vi "pid analog.vi"() -> ()   [LabVIEW 2015]
uses:
  <vilib>/addons/control/pid/pid.llb/PID Control Input Filter (DBL).vi
  <vilib>/addons/control/pid/pid.llb/PID (DBL).vi
  <vilib>/addons/control/pid/pid.llb/PID Output Rate Limiter (DBL).vi
  <vilib>/addons/control/pid/NI_PID_pid.lvlib
panel:
  in  "Array":dbl[](array[numeric])
  in  "Slide 2":dbl(slide) scale=0.0..10.0
  out "Waveform Chart":T1(graph)
  in  "stop":bool
  in  "output rate (EGU/min)":dbl=1.0 format="%.2f"
  in  "dt (s)":dbl=-1.0 format="%.3f"
  # "e"
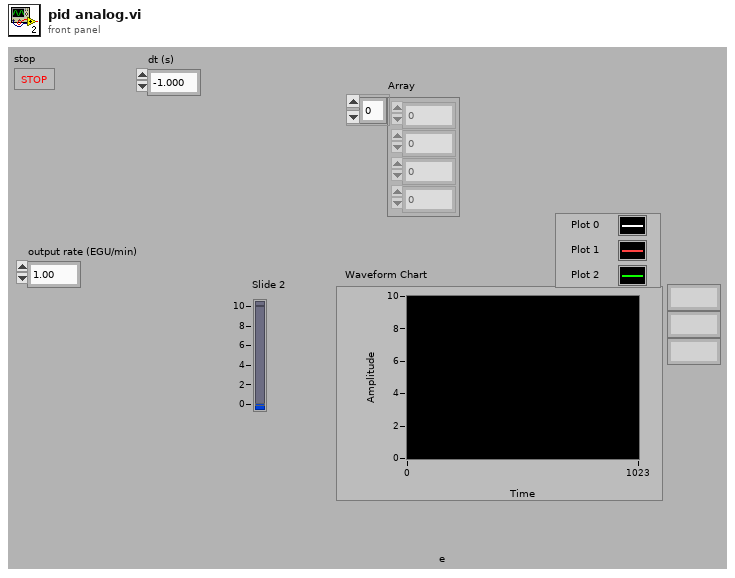
[diagram p1: front panel]
types:
  T1 = cluster{"Slide":dbl, "output":dbl, "Slide 2":dbl}
  T2 = cluster{"Numeric":dbl, "Numeric":dbl, "Numeric":dbl}
  T3 = cluster{"Numeric":dbl, "output":dbl, "output":dbl}
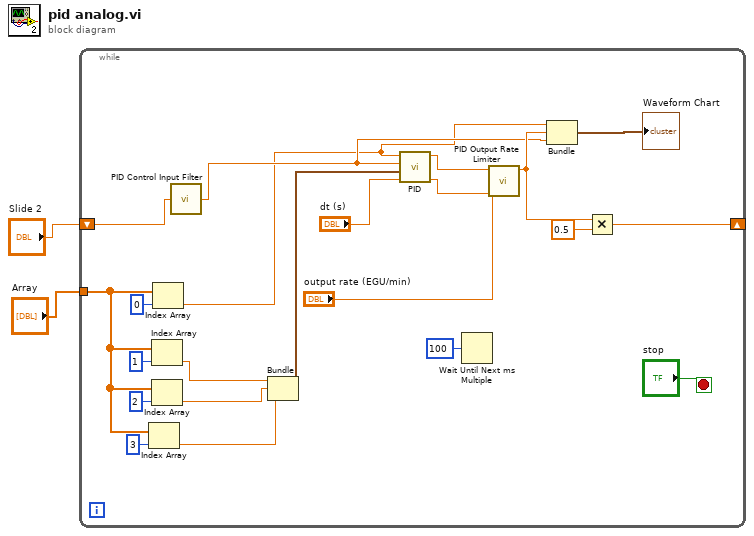
[diagram p0: block diagram]
diagram:
  n1 = while {
    shift-right: [w16] -> _
    shift-left: "Slide 2" -> [w14]
    tunnel: "Array" -> [w10]
    stop <- "stop" stop-if-true
    n2 = Index Array(array=w10, index=3) -> (element=w4:dbl)
    n3 = Index Array(array=w10, index=1) -> (element=w6:dbl)
    n4 = Index Array(array=w10, index=2) -> (element=w5:dbl)
    n5 = Index Array(array=w10, index=0) -> (element=w11:dbl)
    n6 = call-poly <vilib>:"PID Control Input Filter.vi"("input"=w14) -> ("output"=w13:dbl)  [unwired: 4 in]
    n7 = Bundle("Numeric"=w6, "Numeric"=w5, "Numeric"=w4) -> (w3:T2)  [unwired: 1 in]
    n8 = call-poly <vilib>:"PID.vi"("dt (s)"="dt (s)", "PID gains"=w3, "process variable"=w13, "setpoint"=w11) -> ("dt out (s)"=w21:dbl, "output"=w23:dbl)  [unwired: 6 in]
    n9 = Wait Until Next ms Multiple(millisecond multiple=u32 100) -> ()  [unwired: 1 out]
    n10 = call-poly <vilib>:"PID Output Rate Limiter.vi"("dt (s)"=w21, "output rate (EGU/min)"="output rate (EGU/min)", "input (controller output)"=w23) -> ("output"=w18:dbl)  [unwired: 5 in, 1 out]
    n11 = Bundle("Numeric"=w11, "output"=w18, "output"=w13) -> (→"Waveform Chart":T3)  [unwired: 1 in]
    n12 = Multiply(x=w18, y=0.5) -> (x*y=w16:dbl)
  }
